vi "Create Abstract Message for Actor.vi"(7 "Abstract Message Scripter":refnum<class "Abstract Message Scripter.lvclass">, 8 "error in (no error)":errorcluster, 11 "Object":T1) -> (0 "error out":errorcluster)   [LabVIEW 2020, in "Actor Message Maker Provider.lvlib"]
uses:
  Actor Message Maker Provider.lvlib
  MessageMakerProvider/_Message Maker/_Maker Classes/User Defined Prototype/User Defined Prototype.lvclass
  MessageMakerProvider/_Message Maker/_Maker Classes/Message Scripter/Message Scripter.lvclass
  MessageMakerProvider/_Message Maker/_Maker Classes/Reference Method Prototyper/Reference Method Prototyper.lvclass
  MessageMakerProvider/_Message Maker/_Maker Classes/Concrete Send Renamer/Concrete Send Renamer.lvclass
  MessageMakerProvider/_Message Maker/_Maker Classes/Abstract Message Scripter/Abstract Message Scripter.lvclass
  MessageMakerProvider/AFPP Shared/AFPP Shared.lvlib
  <vilib>/ErrorRing/Error Ring.xnode
  MessageMakerProvider/AFPP Shared/Validation Mode.ctl
  <vilib>/Utility/error.llb/Error Cluster From Error Code.vi
  MessageMakerProvider/_Message Maker/_Maker Classes/Abstract Icon Prototyper/Abstract Icon Prototyper.lvclass
  <resource>/Framework/Providers/API/ItemRef.ctl
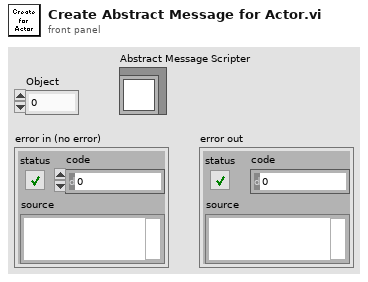
[diagram p1: front panel]
types:
  T1 = typedef "ItemRef.ctl" = u64
  T2 = typedef "AFPP Shared.lvlib/Validation Mode.ctl" = enum16{"An Actor Library", "A Target Tag"}
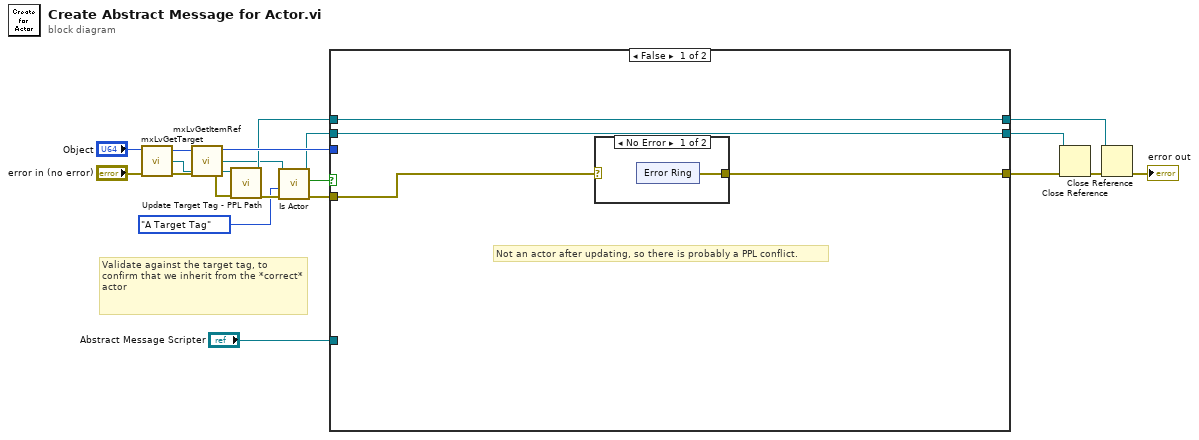
[diagram p0: block diagram]
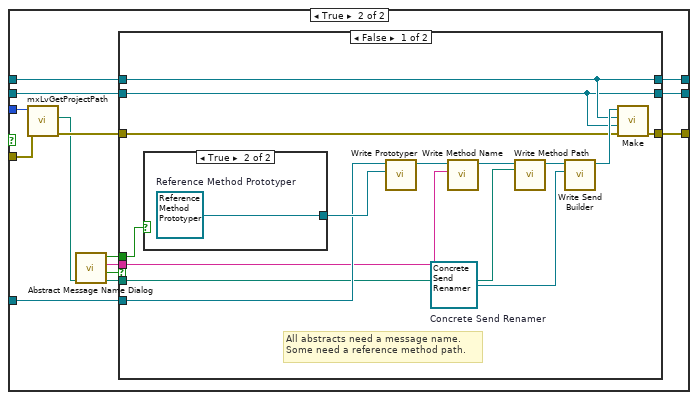
[diagram p3: hidden frame]
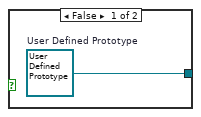
[diagram p4: hidden frame]
diagram:
  # "Validate against the target tag, to confirm that we inherit from the *correct* actor"
  n1 = call <resource>:"mxLvGetTarget.vi"("Item"="Object", "error in"="error in (no error)") -> ("Item"=w18:T1, "Target"=w11:refnum<vi>, "error out"=w17:errorcluster)
  n2 = call <resource>:"mxLvGetItemRef.vi"("Item"=w18, "error in"=w17) -> ("Item"=w14:T1, "Item Refnum"=w9:refnum<vi>, "error out"=w13:errorcluster)
  n3 = call "Update Target Tag - PPL Path.vi"("error in (no error)"=w13, "Target"=w11) -> ("error out"=w12:errorcluster, "dup Target"=w10:refnum<vi>)  [unwired: 7 in, 1 out]
  n4 = call "Is Actor.vi"("error in (no error)"=w12, "Validation"=Validation_Mode."A Target Tag", "ProjectItem in"=w9) -> ("error out"=w2:errorcluster, "Is Actor"=w3:bool, "ProjectItem out"=w8:refnum<vi>)  [unwired: 4 in, 2 out]
  n5 = case shown="False" w3 {
    tunnel: [w22 w45] -> w20
    tunnel: "Abstract Message Scripter" -> [_ w41]
    tunnel: w14 -> [_ w37]
    tunnel: w10 -> [w24 w36]
    tunnel: w8 -> [w23 w35]
    tunnel: [w24 w34] -> w5
    tunnel: [w23 w33] -> w4
    tunnel: w2 -> [w21 w32]
    frame False {
      # "Not an actor after updating, so there is probably a PPL conflict."
      n6 = case shown="No Error" w21 {
        selector: w21 -> [_ w31]
        tunnel: [w25 w31] -> w22
        frame No Error {
          n7 = xnode "Error Ring"() -> ("error out"=w25:errorcluster)
        }
        frame Error {
        }
      }
    }
    frame True {
      n8 = call <resource>:"mxLvGetProjectPath.vi"("error in"=w32, "Item"=w37) -> ("error out"=w40:errorcluster, "Project Path"=w39:path)  [unwired: 7 in, 1 out]
      n9 = call "Abstract Message Name Dialog.vi"("Start Path"=w39) -> ("Path out"=w38:path, "Cancelled?"=w44:bool, "Name"=w43:string, "Use Reference Method out"=w42:bool)  [unwired: 7 in]
      n10 = case shown="False" w44 {
        tunnel: w40 -> [w55 w64]
        tunnel: [w46 w64] -> w45
        tunnel: w43 -> [w52 _]
        tunnel: w42 -> [w57 _]
        tunnel: w41 -> [w56 _]
        tunnel: w38 -> [w49 _]
        tunnel: w36 -> [w48 w63]
        tunnel: w35 -> [w47 w62]
        tunnel: [w48 w63] -> w34
        tunnel: [w47 w62] -> w33
        frame False {
          w54 = refnum<class "Concrete Send Renamer.lvclass"> refnum  # Concrete Send Renamer
          # "All abstracts need a message name.\nSome need a reference method path."
          n11 = case shown="True" w57 {
            tunnel: [w60 w61] -> w58
            frame False {
              w60 = refnum<class "User Defined Prototype.lvclass"> refnum  # User Defined Prototype
            }
            frame True {
              w61 = refnum<class "Reference Method Prototyper.lvclass"> refnum  # Reference Method Prototyper
            }
          }
          n12 = call "Write Prototyper.vi"("Prototyper"=w58, "Message Scripter in"=w56) -> ("Message Scripter out"=w53:refnum<class "Abstract Message Scripter.lvclass">)  [unwired: 9 in]
          n13 = call "Write Method Name.vi"("Method Name"=w52, "Abstract Message Scripter in"=w53) -> ("Abstract Message Scripter out"=w51:refnum<class "Abstract Message Scripter.lvclass">)  [unwired: 9 in]
          n14 = call "Write Method Path.vi"("Method Path"=w49, "Message Scripter in"=w51) -> ("Message Scripter out"=w50:refnum<class "Abstract Message Scripter.lvclass">)  [unwired: 9 in]
          n15 = call "Write Send Builder.vi"("Message Maker.lvlib:Send Builder.lvclass"=w54, "Message Scripter in"=w50) -> ("Message Scripter out"=w59:refnum<class "Abstract Message Scripter.lvclass">)  [unwired: 9 in]
          n16 = call-dynamic "Make.vi"("error in (no error)"=w55, "Item Refnum"=w47, "Target"=w48, "Abstract Message Scripter"=w59) -> ("error out"=w46:errorcluster)  [unwired: 6 in, 1 out]
        }
        frame True {
        }
      }
    }
  }
  n17 = Close Reference(reference=w4, error in (no error)=w20) -> (error out=w6:errorcluster)
  n18 = Close Reference(reference=w5, error in (no error)=w6) -> (error out=→"error out":errorcluster)
